vi "Solve2.vi"(8 "Error In":errorcluster, 11 "object in":refnum<class "2024_9.lvclass">) -> (0 "Error Out":errorcluster, 2 "Result":u64, 3 "object out":refnum<class "2024_9.lvclass">)   [LabVIEW 2023, in "2024_9.lvclass"]
uses:
  2024_9.lvclass
  2024_9.lvclass/2024_9.ctl
panel:
  out "FileData":u8[](array[numeric])
  out "DiscData":i64[](array[numeric])
  out "FileStartIndexOnDisc":i32[](array[numeric])
  out "string 2":string
  out "string":string
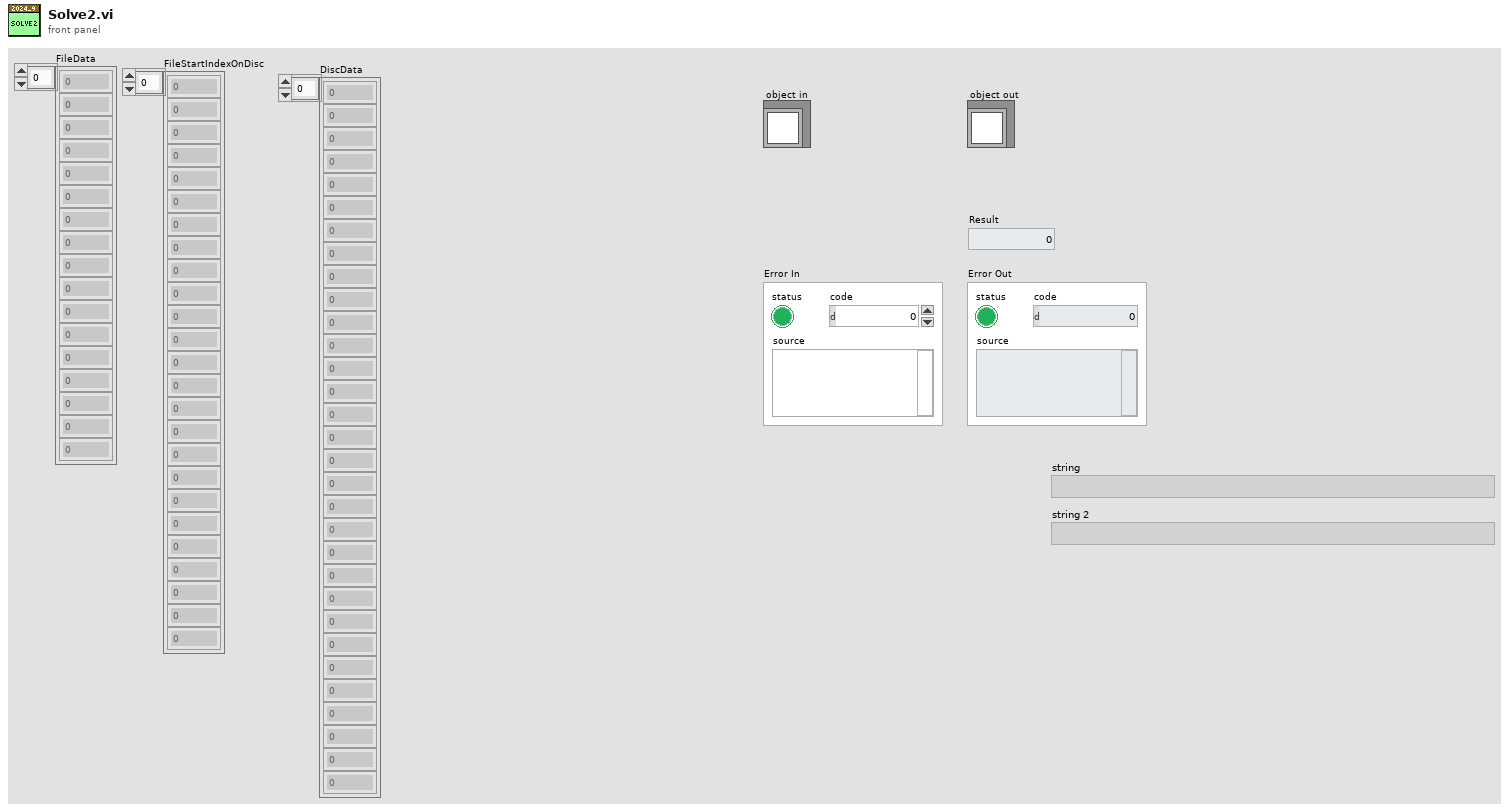
[diagram p1: front panel]
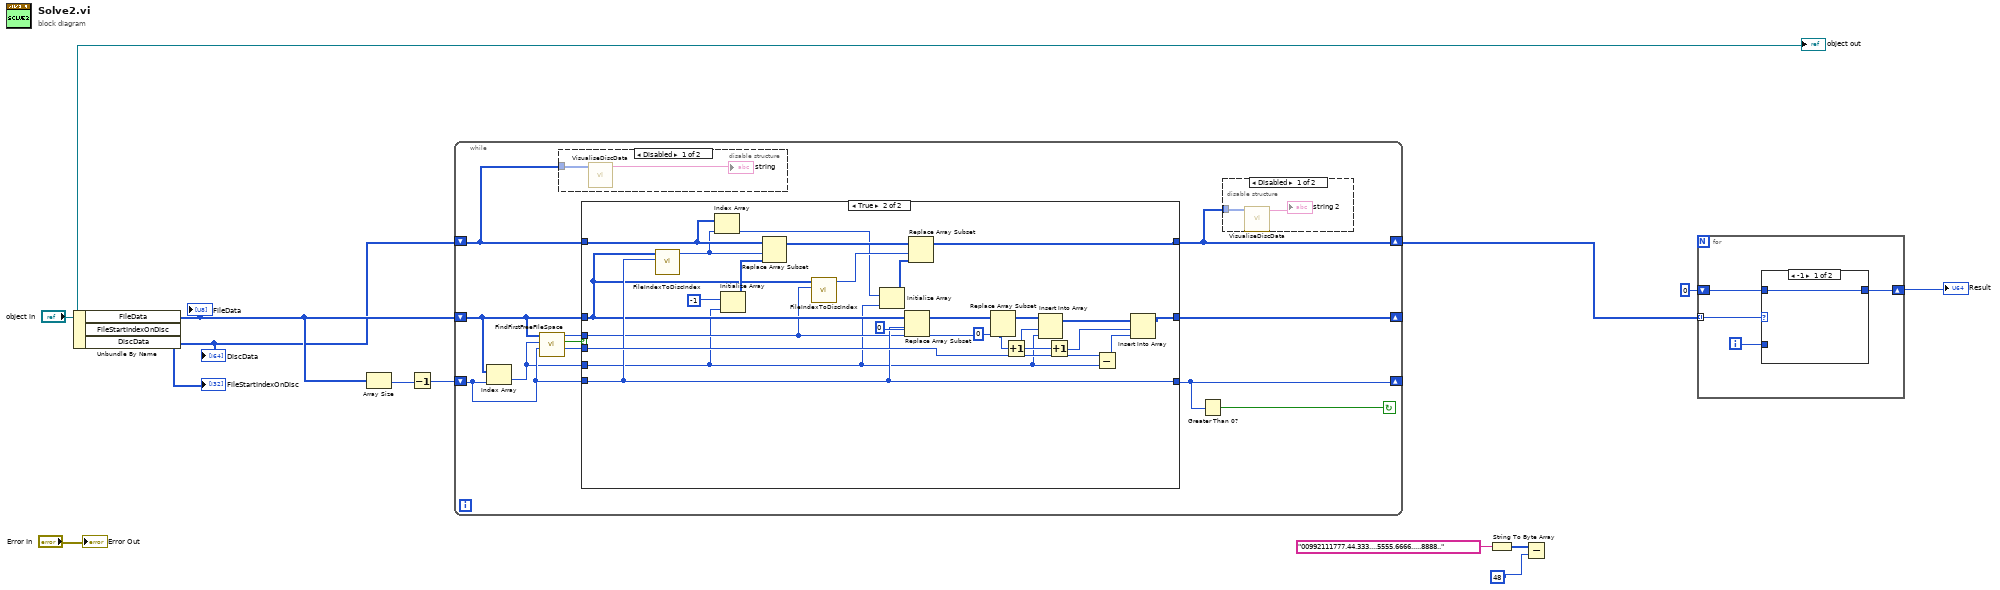
[diagram p0: block diagram]
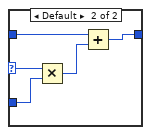
[diagram p2: hidden frame]
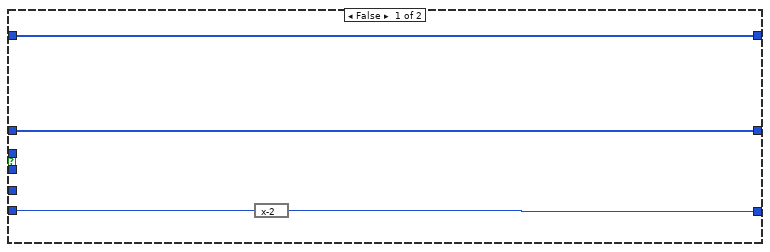
[diagram p5: hidden frame]
diagram:
  n1 = Unbundle By Name("object in") -> ("FileData"=w8:u8[], "FileStartIndexOnDisc"=→"FileStartIndexOnDisc":i32[], "DiscData"=w3:i64[])
  "DiscData" <- w3
  "FileData" <- w8
  n2 = Array Size(array=w8) -> (size(s)=w10:i32)
  n3 = Decrement(x=w10) -> (x-1=w9:i32)
  n4 = while {
    shift-right: [w20] -> _
    shift-left: w8 -> [w16]
    shift-right: [w22] -> _
    shift-left: w9 -> [w23]
    shift-right: [w15] -> w2
    shift-left: w3 -> [w14]
    stop <- w21 continue-if-true
    n5 = Index Array(array=w16, index=w23) -> (element=w18:u8)
    n6 = call "FindFirstFreeFIleSpace.vi"("MaxSearchIndex"=w23, "FileSize"=w18, "FileData"=w16) -> ("ValueOfFreeSpace(Size)"=w17:u8, "FreeSpaceFound"=w24:bool, "IndexOfFirstFreeDiscSpace"=w19:i32)  [unwired: 6 in]
    n7 = disable-structure shown="Disabled" {
      disable-tunnel: w14 -> [w27 _]
      frame Disabled {
        n8 = call "VisualiseDiscData.vi"("DiscData"=w27) -> ("result string"=→"string":string)  [unwired: 10 in]
      }
      frame Enabled {
      }
    }
    n9 = case shown="True" w24 {
      tunnel: w16 -> [w32 w42]
      tunnel: [w32 w48] -> w20
      tunnel: w23 -> [w31 w45]
      tunnel: [w30 w45] -> w22
      tunnel: w19 -> [_ w41]
      tunnel: w18 -> [_ w37]
      tunnel: w17 -> [_ w50]
      tunnel: w14 -> [w29 w35]
      tunnel: [w29 w39] -> w15
      frame False {
        n10 = expression code="x-2"(w31) -> (w30:i32)
      }
      frame True {
        n11 = call "FileIndexToDiscIndex.vi"("FileIndex"=w45, "FileData"=w42) -> ("DiscIndees"=w34:u64)  [unwired: 9 in]
        n12 = Index Array(array=w35, index=w34) -> (element=w33:i64)
        n13 = Initialize Array(i64 -1, w37) -> (w43:i64[])
        n14 = Replace Array Subset(array=w35, new element=w43, index=w34) -> (w40:i64[])
        n15 = call "FileIndexToDiscIndex.vi"("FileIndex"=w41, "FileData"=w42) -> ("DiscIndees"=w38:u64)  [unwired: 9 in]
        n16 = Initialize Array(w33, w37) -> (w36:i64[])
        n17 = Replace Array Subset(array=w42, new element=u8 0 ("new element/subarray"), index=w45) -> (w47:u8[])
        n18 = Replace Array Subset(array=w40, new element=w36, index=w38) -> (w39:i64[])
        n19 = Replace Array Subset(array=w47, new element=u8 0 ("new element/subarray"), index=w41) -> (w54:u8[])
        n20 = Increment(x=w41) -> (x+1=w52:i32)
        n21 = Insert Into Array(array=w54, index=w52, new element=w37) -> (w53:u8[])
        n22 = Increment(x=w52) -> (x+1=w51:i32)
        n23 = Subtract(x=w50, y=w37) -> (x-y=w49:u8)
        n24 = Insert Into Array(array=w53, index=w51, new element=w49) -> (w48:u8[])
      }
    }
    n25 = Greater Than 0?(x=w22) -> (x > 0?=w21:bool)
    n26 = disable-structure shown="Disabled" {
      disable-tunnel: w15 -> [w25 _]
      frame Disabled {
        n27 = call "VisualiseDiscData.vi"("DiscData"=w25) -> ("result string"=→"string 2":string)  [unwired: 10 in]
      }
      frame Enabled {
      }
    }
  }
  n28 = String To Byte Array(string="00992111777.44.333....5555.6666.....8888..") -> (unsigned byte array=w6:u8[])
  n29 = Subtract(x=w6, y=48) -> ()  [unwired: 1 out]
  n30 = for {
    tunnel: w2 -> [w59] mode=indexing
    shift-right: [w56] -> w12
    shift-left: u64 0 -> [w57]
    i -> [w58]
    n31 = case shown="-1" w59 {
      selector: w59 -> [_ w65]
      tunnel: w58 -> [_ w64]
      tunnel: w57 -> [w60 w62]
      tunnel: [w60 w61] -> w56
      frame -1 {
      }
      frame Default {
        n32 = Multiply(x=w65, y=w64) -> (x*y=w63:i64)
        n33 = Add(x=w62, y=w63) -> (x+y=w61:u64)
      }
    }
  }
  "Result" <- w12
  "Error Out" <- "Error In"
  "object out" <- "object in"
